vi "Decode PNG tIMe Chunk.vi"(10 "error in (no error)":errorcluster, 11 "data":u8[](array[numeric])) -> (2 "error out":errorcluster, 3 "Time Last Modified":T1)   [LabVIEW 2021, in "Files.lvlib"]
uses:
  Files.lvlib
  PNG Time Last Modified.ctl
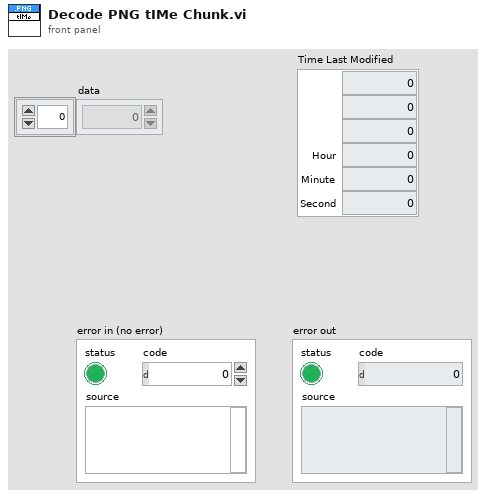
[diagram p1: front panel]
types:
  T1 = typedef "Files.lvlib/PNG Time Last Modified.ctl" = cluster{"Year":u16, "Month":u8, "Day":u8, "Hour":u8, "Minute":u8, "Second":u8}
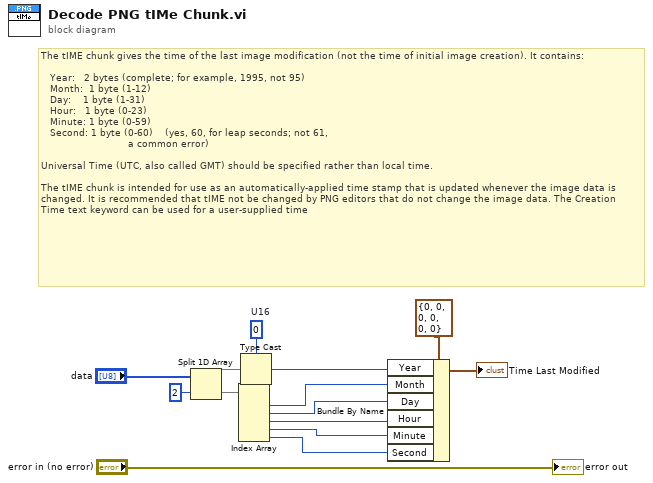
[diagram p0: block diagram]
diagram:
  w9 = u16 0  # U16
  # "The tIME chunk gives the time of the last image modification (not the time of initial image creation). It contains:\n\n   Year:   2 bytes (complete; for example, 1995, not 95)\n   Month:  1 byte (1-12)\n   Day:    1 byte (1-31)\n   Hour:   1 byte (0-23)\n   Minute: 1 byte (0-59)\n   Second: 1 byte (0-60)    (yes, 60, for leap seconds; not 61,\n                             a common error)\n\nUniversal Time (UTC, also called GMT) should be specified rather than local time.\n\nThe tIME chunk is intended for use as an automatically-applied time stamp that is updated whenever the image data is changed. It is recommended that tIME not be changed by PNG editors that do not change the image data. The Creation Time text keyword can be used for a user-supplied time"
  n1 = Split 1D Array(array="data", index=2) -> (first subarray=w10:u8[], second subarray=w12:u8[])
  n2 = Index Array(array=w12) -> (element #1=w5:u8, element #2=w4:u8, element #3=w3:u8, element #4=w2:u8, element #5=w1:u8)  [unwired: 5 in]
  n3 = Type Cast(type=w9, x=w10) -> (*(type *) &x=w8:u16)
  n4 = Bundle By Name(cluster=T1 {"Year"=0, "Month"=0, "Day"=0, "Hour"=0, "Minute"=0, "Second"=0} ("Time Last Modified"), "Year"=w8, "Month"=w5, "Day"=w4, "Hour"=w3, "Minute"=w2, "Second"=w1) -> (→"Time Last Modified":T1)
  "error out" <- "error in (no error)"
